vi "B7_72_82_StandartRangeSelect (SubVI).vi"(1 "Control Point":dbl, 2 "RangeDigit":dbl[](array[numeric]), 4 "RangeCommand":string[](array[string])) -> (0 "R/O":string)   [LabVIEW 2018]
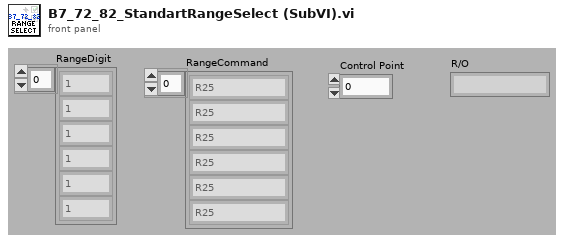
[diagram p1: front panel]
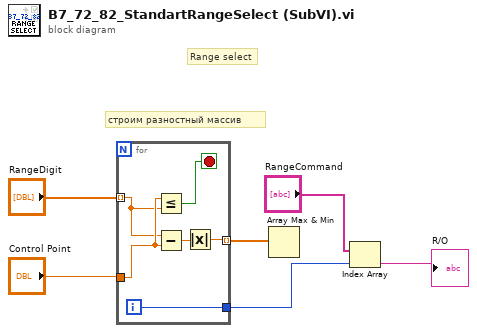
[diagram p0: block diagram]
diagram:
  # "строим разностный массив"
  # "Range select"
  n1 = for {
    tunnel: "RangeDigit" -> [w8] mode=indexing
    tunnel: "Control Point" -> [w9]
    tunnel: [w11] -> w4 mode=indexing
    tunnel: [w10] -> w1
    i -> [w10]
    stop <- w7 stop-if-true
    n2 = Less Or Equal?(x=w9, y=w8) -> (x <= y?=w7:bool)
    n3 = Subtract(x=w8, y=w9) -> (x-y=w12:dbl)
    n4 = Absolute Value(x=w12) -> (abs(x)=w11:dbl)
  }
  n5 = Array Max & Min(array=w4) -> ()  [unwired: 4 out]
  n6 = Index Array(array="RangeCommand", index=w1) -> (element=→"R/O":string)
